vi "1.2.vi"() -> ()   [LabVIEW 2020]
panel:
  in  "String":string
  out "String":string
  out "Thermometer":dbl(slide) scale=0.0..100.0
  in  "DBL":dbl(knob) scale=0.0..100.0
  out "boleano":bool
  out "INT":i32
  in  "INT":i32
  in  "boleano":bool
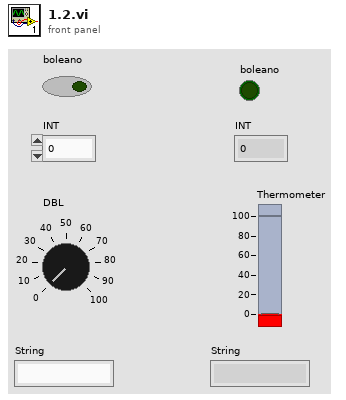
[diagram p1: front panel]
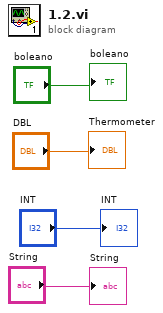
[diagram p0: block diagram]
diagram:
  "INT" <- "INT"
  "boleano" <- "boleano"
  "Thermometer" <- "DBL"
  "String" <- "String"
